vi "ReadIOConfig.vi"(8 "error in (no error)":errorcluster) -> (0 "error out":errorcluster, 3 "DioConfig":string[][](array[string]))   [LabVIEW 2009]
uses:
  <vilib>/Utility/file.llb/Read From Spreadsheet File (string).vi
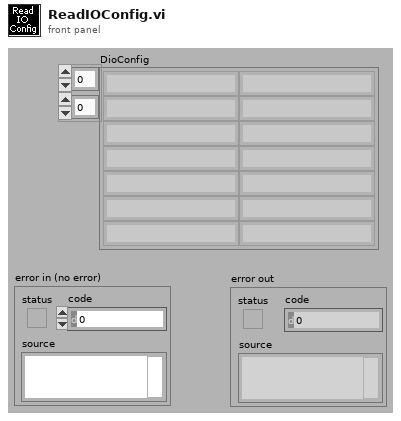
[diagram p1: front panel]
types:
  T1 = enum32{"invalid app kind", "Development System", "Run Time System", "Student Edition", "Embedded LabVIEW", "Evaluation", "Custom"}
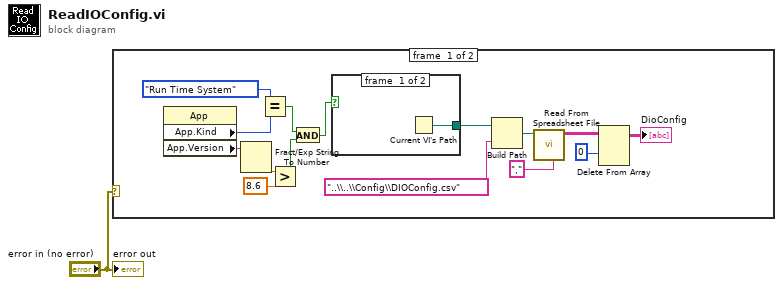
[diagram p0: block diagram]
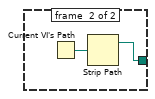
[diagram p2: hidden frame]
diagram:
  n1 = case shown="No Error" "error in (no error)" {
    frame #0 {
      n2 = property class="App"() -> ("App.Kind"=w4:T1, "App.Version"=w5:string)  [unwired: 2 in, 2 out]
      n3 = Fract/Exp String To Number(string=w5) -> (number=w6:dbl)  [unwired: 4 out]
      n4 = Equal?(x=T1."Run Time System" ("y"), y=w4) -> (x = y?=w8:bool)
      n5 = Greater?(x=w6, y=8.6) -> (0:w9:bool)
      n6 = And(x=w8, y=w9) -> (x .and. y?=w2:bool)
      n7 = case shown="True" w2 {
        tunnel: [w17 w19] -> w15
        frame #0 {
          n8 = Current VI's Path() -> (path=w17:path)
        }
        frame #1 {
          n9 = Current VI's Path() -> (path=w18:path)
          n10 = Strip Path(path=w18) -> (stripped path=w19:path)  [unwired: 1 out]
        }
      }
      n11 = Build Path(base path=w15, name or relative path="..\\..\\Config\\DIOConfig.csv" ("名称或相对路径")) -> (appended path=w14:path)
      n12 = call-poly <vilib>:"Read From Spreadsheet File.vi"("delimiter (\\t)"="," ("delimiter (\\t)"), "file path (dialog if empty)"=w14) -> ("all rows"=w11:string[][])  [unwired: 3 in, 6 out]
      n13 = Delete From Array(array=w11, index (row)=0) -> (array with subset deleted=→"DioConfig":string[][])  [unwired: 2 in, 1 out]
    }
    frame #1 {
    }
  }
  "error out" <- "error in (no error)"
